vi "Action Name.vi"(11 "UpdateAction in":refnum<class "DependAction.lvclass">) -> (2 "Action Name":string)   [LabVIEW 2020, in "GPackTools.lvlib" / "DependAction.lvclass"]
uses:
  DependAction.lvclass
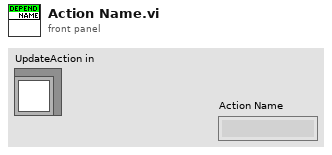
[diagram p1: front panel]
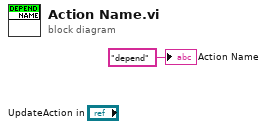
[diagram p0: block diagram]
diagram:
  "Action Name" <- "depend" ("Action Name")
